vi "Update Info.vi"(8 "error in (no error)":errorcluster, 10 "Vecto Info":T1, 11 "VectoService in":refnum<class "VectoInfo.lvclass">) -> (0 "error out":errorcluster, 3 "VectoService out":refnum<class "VectoInfo.lvclass">)   [LabVIEW 2020, in "Vecto.lvlib" / "VectoInfo.lvclass"]
uses:
  VectoInfo.lvclass
  Vecto Info.ctl
  Connection Info.ctl
  Connection Type.ctl
  Info Data.ctl
  VectoInfo.lvclass/VectoInfo.ctl
  Vecto.lvlib
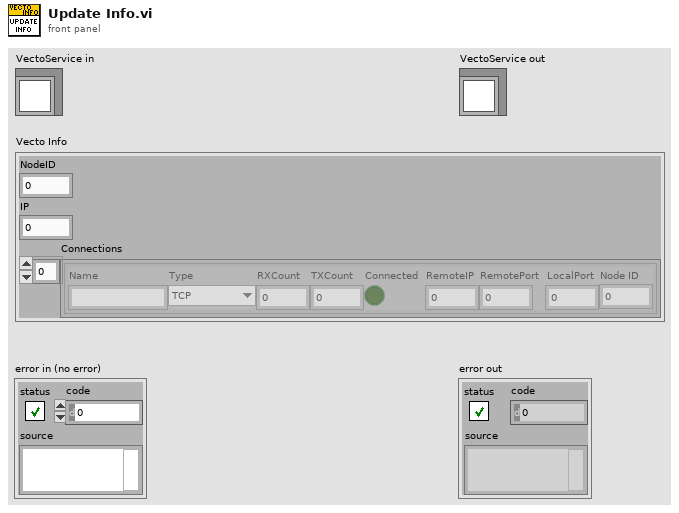
[diagram p1: front panel]
types:
  T1 = typedef "Vecto.lvlib/Vecto Info.ctl" = cluster{"NodeID":i32, "IP":u32, "Connections":T2[]}
  T2 = typedef "Vecto.lvlib/Connection Info.ctl" = cluster{"Name":string, "Type":T3, "RXCount":i32, "TXCount":i32, "Connected":bool, "RemoteIP":u32, "RemotePort":u16, "LocalPort":u16, "Node ID":u32}
  T3 = typedef "Vecto.lvlib/Connection Type.ctl" = enum16{"TCP", "Telemetry", "Discovery", "HTTP"}
  T4 = typedef "Vecto.lvlib/VectoInfo.lvclass/Info Data.ctl" = cluster{"Info":T1}
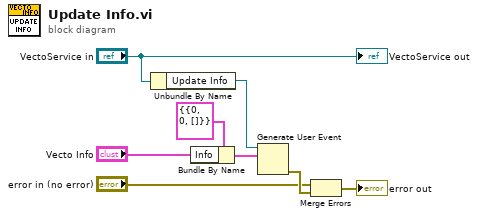
[diagram p0: block diagram]
diagram:
  n1 = Unbundle By Name("VectoService in") -> ("Update Info"=w7:refnum<user-event>)
  n2 = Bundle By Name(cluster=T4 {"Info"={"NodeID"=0, "IP"=0, "Connections"=[]}} ("event data"), "Info"="Vecto Info") -> (w5:T4)
  n3 = Generate User Event(user event=w7, event data cluster=w5) -> (error out=w3:errorcluster)  [unwired: 2 in, 1 out]
  n4 = Merge Errors("error in (no error)", w3) -> (→"error out":errorcluster)
  "VectoService out" <- "VectoService in"
